vi "sub_cam_main.vi"(8 "error in":errorcluster) -> (0 "error out":errorcluster={"status"=FALSE, "code"=1122, "source"=""})   [LabVIEW 2019]
uses:
  <resource>/objmgr/IMAQImage.rc
panel:
  out "n":i32
  out "Image":T1(plugin-control)
  out "loop run":i32=2958
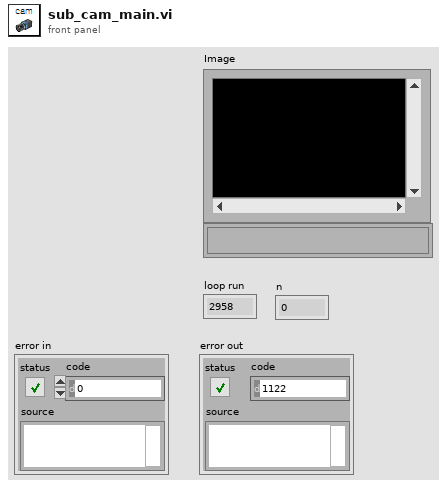
[diagram p1: front panel]
types:
  T1 = typedef "IMAQ Image.ctl" = refnum<image>
  T2 = typedef "control_ref.ctl" = cluster{"VLP16 cfg":refnum<vi>, "TIM571 cfg":refnum<vi>, "PID cfg":refnum<vi>, "AGV cfg":refnum<vi>, "GNSS cfg":refnum<vi>, "camera cfg":refnum<vi>, "ybbaek copyright":refnum<vi>, "Obstacle limit cfg":refnum<vi>, "State machine cfg":refnum<vi>, "Lookahead cfg":refnum<vi>, "waypoint files cfg":refnum<vi>, "Vison cfg":refnum<vi>, "RPLidar cfg":refnum<vi>, "point all":refnum<vi>, "HW info":refnum<vi>, "Joystick cfg":refnum<vi>, "GMapControl":refnum<vi>}
  T3 = cluster{"x-center":dbl, "Image Size":cluster{"x":i32, "y":i32}, "Angle deg":sgl, "Threshold Range":cluster{"Lower value":sgl, "Upper value":sgl}}
  T4 = typedef "status.ctl" = u16
  T5 = cluster{"AGV":T4, "AGV Estop":T4, "Obstacle":T4, "Heading":T4, "Waypt":T4, "GNSS":T4, "VLP16":T4, "Cam":T4, "RPLidar":T4, "Joystick":T4}
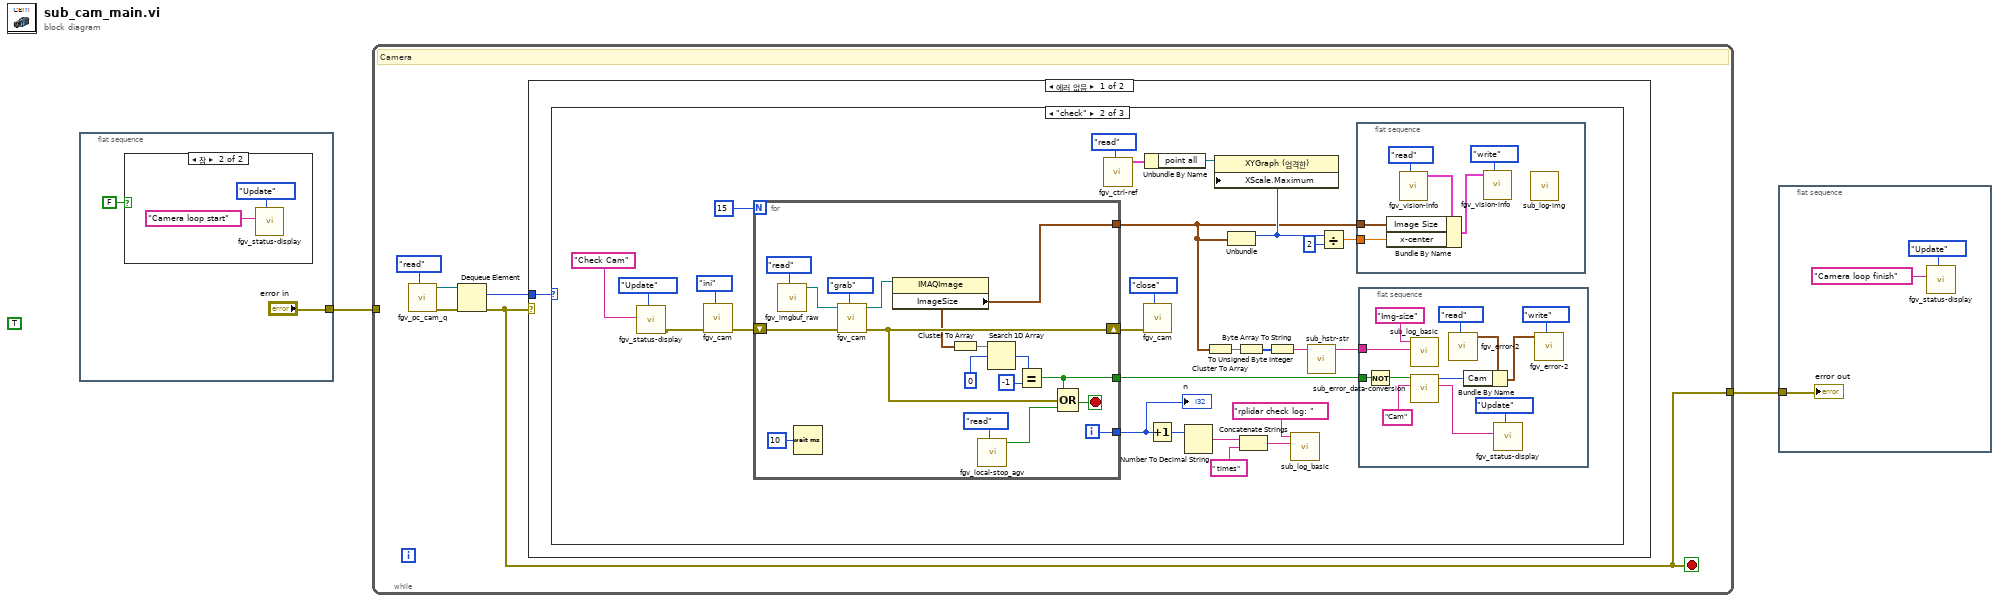
[diagram p0: block diagram]
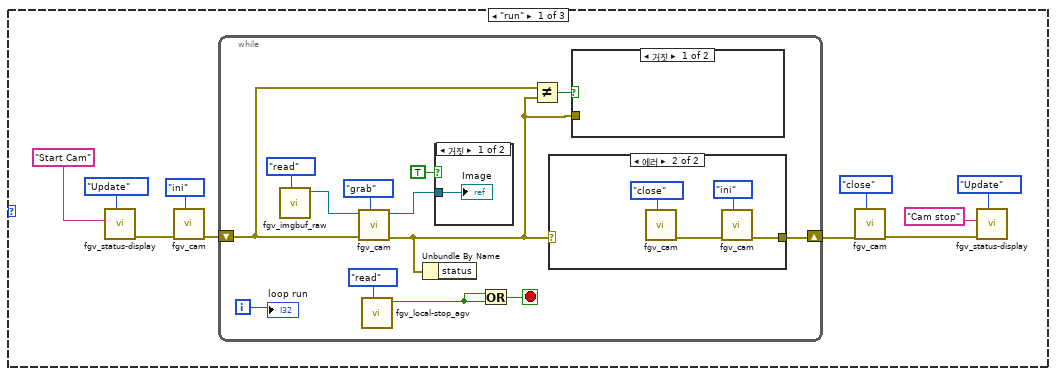
[diagram p3: hidden frame]
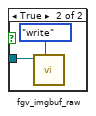
[diagram p5: hidden frame]
diagram:
  (unwired) TRUE
  n1 = flat-sequence {
    tunnel: ["error in"] -> w1
    frame #0 {
      n2 = case shown="참" FALSE {
        frame False {
        }
        frame True {
          n3 = call "fgv_status-display.vi"("Mode"=enum16{"Initial", "Update", "Clear"}."Update", "title"="Camera loop start" ("String in 1")) -> ()  [unwired: 9 in, 1 out]
        }
      }
    }
  }
  n4 = while {
    tunnel: [w7] -> w2
    tunnel: w1 -> [_]
    stop <- w7 stop-if-true
    # "Camera"
    n5 = call "fgv_pc_cam_q.vi"("cmd"=enum16{"create", "write", "read", "close"}."read") -> ("error out"=w10:errorcluster, "queue out"=w9:refnum<queue>)  [unwired: 9 in]
    n6 = Dequeue Element(queue=w9, error in (no error)=w10) -> (element=w8:enum16{"run", "check", "stop"}, error out=w7:errorcluster)  [unwired: 1 in, 2 out]
    n7 = case shown="에러 없음" w7 {
      tunnel: w8 -> [w12 _]
      frame No Error {
        n8 = case shown="\"check\"" w12 {
          frame "run" {
            n9 = call "fgv_status-display.vi"("Mode"=enum16{"Initial", "Update", "Clear"}."Update", "title"="Start Cam" ("String in")) -> ("error out"=w14:errorcluster)  [unwired: 9 in]
            n10 = call "fgv_cam.vi"("cmd"=enum16{"ini", "grab", "close", "read"}."ini", "error in"=w14) -> ("error out"=w22:errorcluster)  [unwired: 7 in, 2 out]
            n11 = while {
              shift-right: [w32] -> w21
              shift-left: w22 -> [w25]
              i -> [w29]
              stop <- w35 stop-if-true
              n12 = call "fgv_imgbuf_raw.vi"("cmd"=enum16{"create", "close", "write", "read"}."read") -> ("Image"=w34:T1)  [unwired: 9 in, 1 out]
              n13 = call "fgv_cam.vi"("cmd"=enum16{"ini", "grab", "close", "read"}."grab", "error in"=w25, "Image In"=w34) -> ("error out"=w23:errorcluster, "Image Out"=w26:T1)  [unwired: 6 in, 1 out]
              n14 = call "fgv_local-stop_agv.vi"("cmd"=enum16{"ini", "read", "stop"}."read") -> ("stop status"=w30:bool)  [unwired: 10 in]
              n15 = Unbundle By Name(w23) -> ()  [unwired: 1 out]
              n16 = case shown="거짓" TRUE {
                tunnel: w26 -> [w36 w37]
                frame False {
                  "Image" <- w36
                }
                frame True {
                  n17 = call "fgv_imgbuf_raw.vi"("cmd"=enum16{"create", "close", "write", "read"}."write", "raw Image in"=w37) -> ()  [unwired: 8 in, 2 out]
                }
              }
              n18 = Or(x=w30, y=w30) -> (x .or. y?=w35:bool)
              n19 = Not Equal?(x=w25, y=w23) -> (x != y?=w24:bool)
              n20 = case shown="에러" w23 {
                selector: w23 -> [w39 _]
                tunnel: [w39 w42] -> w32
                frame No Error {
                }
                frame Error {
                  n21 = call "fgv_cam.vi"("cmd"=enum16{"ini", "grab", "close", "read"}."close") -> ("error out"=w43:errorcluster)  [unwired: 8 in, 2 out]
                  n22 = call "fgv_cam.vi"("cmd"=enum16{"ini", "grab", "close", "read"}."ini", "error in"=w43) -> ("error out"=w42:errorcluster)  [unwired: 7 in, 2 out]
                }
              }
              n23 = case shown="거짓" w24 {
                tunnel: w23 -> [_ _]
                frame False {
                }
                frame True {
                }
              }
              "loop run" <- w29
            }
            n24 = call "fgv_cam.vi"("cmd"=enum16{"ini", "grab", "close", "read"}."close", "error in"=w21) -> ("error out"=w18:errorcluster)  [unwired: 7 in, 2 out]
            n25 = call "fgv_status-display.vi"("Mode"=enum16{"Initial", "Update", "Clear"}."Update", "error in"=w18, "title"="Cam stop" ("String in")) -> ()  [unwired: 8 in, 1 out]
          }
          frame "check" {
            n26 = call "fgv_status-display.vi"("Mode"=enum16{"Initial", "Update", "Clear"}."Update", "title"="Check Cam" ("String in")) -> ("error out"=w62:errorcluster)  [unwired: 9 in]
            n27 = call "fgv_cam.vi"("cmd"=enum16{"ini", "grab", "close", "read"}."ini", "error in"=w62) -> ("error out"=w69:errorcluster)  [unwired: 7 in, 2 out]
            n28 = for {
              N: 15 -> [_]
              shift-right: [w97] -> w55
              shift-left: w69 -> [w104]
              tunnel: [w98] -> w50
              tunnel: [w88] -> w46
              tunnel: [w90] -> w45
              i -> [w98]
              stop <- w95 stop-if-true
              n29 = call "fgv_imgbuf_raw.vi"("cmd"=enum16{"create", "close", "write", "read"}."read") -> ("Image"=w103:T1)  [unwired: 9 in, 1 out]
              n30 = Wait (ms)(milliseconds to wait=u32 10) -> ()  [unwired: 1 out]
              n31 = call "fgv_cam.vi"("cmd"=enum16{"ini", "grab", "close", "read"}."grab", "error in"=w104, "Image In"=w103) -> ("error out"=w97:errorcluster, "Image Out"=w94:T1)  [unwired: 6 in, 1 out]
              n32 = property class="IMAQImage"(reference=w94) -> ("ImageSize"=w90:cluster{"x":i32, "y":i32})  [unwired: 1 in, 2 out]
              n33 = Cluster To Array(cluster=w90) -> (array=w93:i32[])
              n34 = call "fgv_local-stop_agv.vi"("cmd"=enum16{"ini", "read", "stop"}."read") -> ("stop status"=w96:bool)  [unwired: 10 in]
              n35 = Search 1D Array(1D array=w93, element=0 ("시작 인덱스(0)")) -> (index of element=w92:i32)  [unwired: 1 in]
              n36 = Equal?(x=w92, y=-1) -> (x = y?=w88:bool)
              n37 = Compound Arithmetic op=OR ("복합 연산")(w88, w97, w96) -> (w95:bool)
            }
            "n" <- w50
            n38 = call "fgv_ctrl-ref.vi"("cmd"=enum16{"write", "read"}."read") -> ("ref out"=w60:T2)  [unwired: 9 in, 1 out]
            n39 = call "fgv_cam.vi"("cmd"=enum16{"ini", "grab", "close", "read"}."close", "error in"=w55) -> ()  [unwired: 7 in, 3 out]
            n40 = Unbundle By Name(w60) -> ("point all"=w59:refnum<vi>)
            n41 = Increment(x=w50) -> (x+1=w52:i32)
            n42 = Number To Decimal String(number=w52) -> (decimal integer string=w53:string)  [unwired: 1 in]
            n43 = Cluster To Array(cluster=w45) -> (array=w58:i32[])
            n44 = Unbundle(w45) -> ("x"=w56:i32)  [unwired: 1 out]
            n45 = property class="XYGraph (엄격한)"(reference=w59, "XScale.Maximum"=w56) -> ()  [unwired: 1 in, 2 out]
            n46 = To Unsigned Byte Integer(number=w58) -> (unsigned 8bit integer=w57:u8[])
            n47 = Concatenate Strings(w53, " times" ("문자열")) -> (w49:string)
            n48 = Byte Array To String(unsigned byte array=w57) -> (string=w54:string)
            n49 = call "sub_log_basic.vi"("desc"=w49, "Title"="rplidar check log: ") -> ()  [unwired: 9 in, 1 out]
            n50 = call "sub_hstr-str.vi"("h-str"=w54) -> ("h2n-str"=w44:string)  [unwired: 10 in]
            n51 = Divide(x=w56, y=2) -> (x/y=w61:dbl)
            n52 = flat-sequence {
              tunnel: w61 -> [w71]
              tunnel: w45 -> [w70]
              frame #0 {
                n53 = call "fgv_vision-info.vi"("cmd"=enum16{"read", "write"}."read") -> ("image info out"=w73:T3)  [unwired: 10 in]
                n54 = Bundle By Name(cluster=w73, "Image Size"=w70, "x-center"=w71) -> (w72:T3)
                n55 = call "fgv_vision-info.vi"("cmd"=enum16{"read", "write"}."write", "image info"=w72) -> ()  [unwired: 9 in, 1 out]
                n56 = call "sub_log-img.vi"() -> ()  [unwired: 11 in, 1 out]
              }
            }
            n57 = flat-sequence {
              tunnel: w46 -> [w79]
              tunnel: w44 -> [w77]
              frame #0 {
                n58 = Not(x=w79) -> (.not. x?=w76:bool)
                n59 = call "sub_log_basic.vi"("desc"=w77, "Title"="Img-size") -> ()  [unwired: 9 in, 1 out]
                n60 = call "sub_error_data-conversion.vi"("name"="Cam", "error status"=w76) -> ("check result string"=w81:string, "error conversion out"=w87:T4)  [unwired: 8 in]
                n61 = call "fgv_error-2.vi"("cmd"=enum16{"init", "read", "write"}."read") -> ("Error cluster out"=w86:T5)  [unwired: 9 in, 1 out]
                n62 = Bundle By Name(cluster=w86, "Cam"=w87) -> (w83:T5)
                n63 = call "fgv_status-display.vi"("Mode"=enum16{"Initial", "Update", "Clear"}."Update", "title"=w81) -> ()  [unwired: 9 in, 1 out]
                n64 = call "fgv_error-2.vi"("cmd"=enum16{"init", "read", "write"}."write", "Error cluster"=w83) -> ()  [unwired: 8 in, 2 out]
              }
            }
          }
          frame "stop", Default {
          }
        }
      }
      frame Error {
      }
    }
  }
  n65 = flat-sequence {
    tunnel: w2 -> [w107]
    frame #0 {
      n66 = call "fgv_status-display.vi"("Mode"=enum16{"Initial", "Update", "Clear"}."Update", "title"="Camera loop finish" ("String in 1")) -> ()  [unwired: 9 in, 1 out]
      "error out" <- w107
    }
  }
